vi "Change Receive Window Size.vi"(5 "Username":string, 6 "Password":string, 7 "Address":string, 8 "Error In":errorcluster) -> (0 "Error Out":errorcluster)   [LabVIEW 2018, in "Tests.lvlib" / "Channel.lvlib"]
uses:
  Channel.lvlib
  <vilib>/addons/_JKI Toolkits/Caraya/classes/Test/Test.lvclass
  <vilib>/addons/_JKI Toolkits/Caraya/classes/Assert/Assert.lvclass
  src/Toolkit/Channel/Channel.lvclass
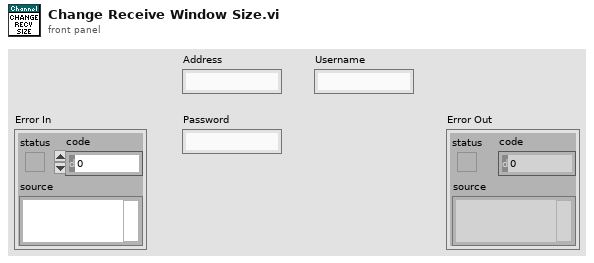
[diagram p1: front panel]
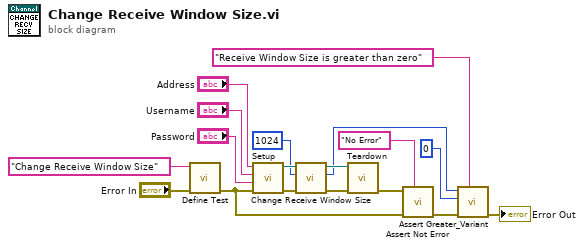
[diagram p0: block diagram]
diagram:
  n1 = call <vilib>:"Define Test.vi"("error in (no error)"="Error In", "Label (VI Title)"="Change Receive Window Size") -> ("error out"=w15:errorcluster)  [unwired: 9 in]
  n2 = call "Setup.vi"("Error In"=w15, "Password"="Password", "Username"="Username", "Address"="Address") -> ("Error Out"=w3:errorcluster, "Channel"=w6:refnum<class "Channel.lvclass">)  [unwired: 6 in]
  n3 = call "Change Receive Window Size.vi"("Error In"=w3, "Size"=u32 1024 ("Adjustment"), "Channel In"=w6) -> ("Error Out"=w4:errorcluster, "Window"=w1:u32, "Channel Out"=w5:refnum<class "Channel.lvclass">)  [unwired: 6 in]
  n4 = call "Teardown.vi"("Error In"=w4, "Channel"=w5) -> ("Error Out"=w11:errorcluster)  [unwired: 9 in]
  n5 = call <vilib>:"Assert Not Error.vi"("Label"="No Error", "error in (no error)"=w15, "Not Error?"=w11) -> ("error out"=w10:errorcluster)  [unwired: 8 in]
  n6 = call <vilib>:"Assert Greater_Variant.vi"("Label"="Receive Window Size is greater than zero", "error in (no error)"=w10, "Y"=u32 0 ("Size"), "X"=w1) -> ("error out"=→"Error Out":errorcluster)  [unwired: 7 in]
